vi "Packager Files Path.vi"(11 "error in (no error)":errorcluster) -> (4 "Template Path":path, 6 "Config File Path":path, 15 "error out":errorcluster)   [LabVIEW 2021, in "Path Functions.lvlib"]
uses:
  Path Functions.lvlib
  <vilib>/Utility/sysdir.llb/System Directory Type.ctl
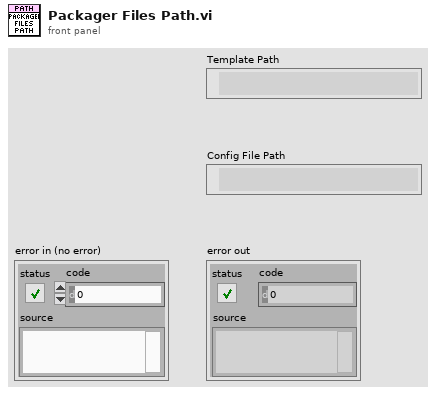
[diagram p1: front panel]
types:
  T1 = typedef "System Directory Type.ctl" = i32
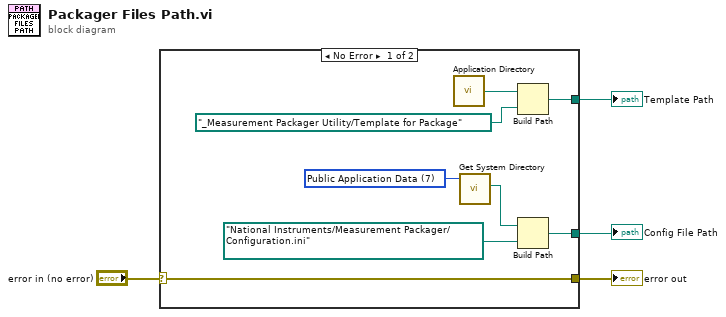
[diagram p0: block diagram]
diagram:
  n1 = case shown="No Error" "error in (no error)" {
    selector: "error in (no error)" -> [w10 w13]
    tunnel: [w12 _] -> w4
    tunnel: [w11 _] -> w3
    tunnel: [w10 w13] -> w2
    frame No Error {
      w6 = T1 7 items=["User Home"=0, "User Desktop"=1, "User Documents"=2, "User Application Data"=3, "User Preferences"=4, "User Temporary"=5, "Public Documents"=6, "Public Application Data"=7, "Public Preferences"=8, "Public Cache"=13, "System Core Libraries"=9, "System Installed Libraries"=10, "Application Files"=11, "Boot Volume Root"=12] ("system directory type")
      n2 = call <vilib>:"Application Directory.vi"() -> ("Application Directory"=w9:path)
      n3 = call <vilib>:"Get System Directory.vi"("system directory type"=w6) -> ("system directory"=w7:path)  [unwired: 10 in]
      n4 = Build Path(base path=w9, name or relative path=path "_Measurement Packager Utility/Template for Package") -> (appended path=w12:path)
      n5 = Build Path(base path=w7, name or relative path=path "National Instruments/Measurement Packager/Configuration.ini") -> (appended path=w11:path)
    }
    frame Error {
    }
  }
  "error out" <- w2
  "Template Path" <- w4
  "Config File Path" <- w3
